vi "Time lapse wait for next frame.vi"(6 "error in (no error)":errorcluster, 8 "Frame Interval (s)":dbl=1.0, 9 "Time of last frame in":u32) -> (0 "error out":errorcluster, 1 "Stopped?":bool, 2 "Sec. till next frame":ext(slide), 3 "Time of this frame out (ms)":u32)   [LabVIEW 2016]
doc: "Waits for the specified time. Used in time-lapse data acquisition."
uses:
  Autofocus Globals.vi
panel:
  in  "Go now":bool
  in  "Pause":bool
  in  "Stop":bool
  # "Parameters not for interactive use"
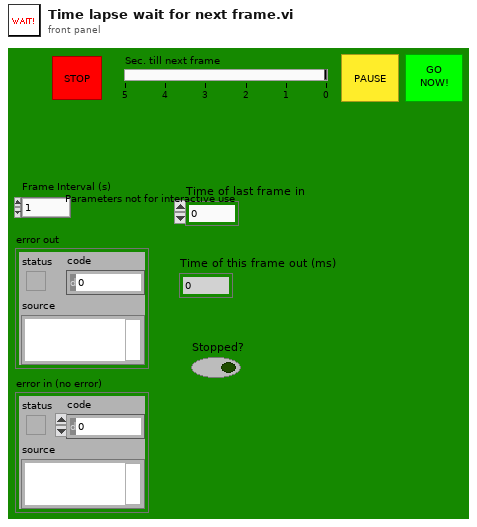
[diagram p1: front panel]
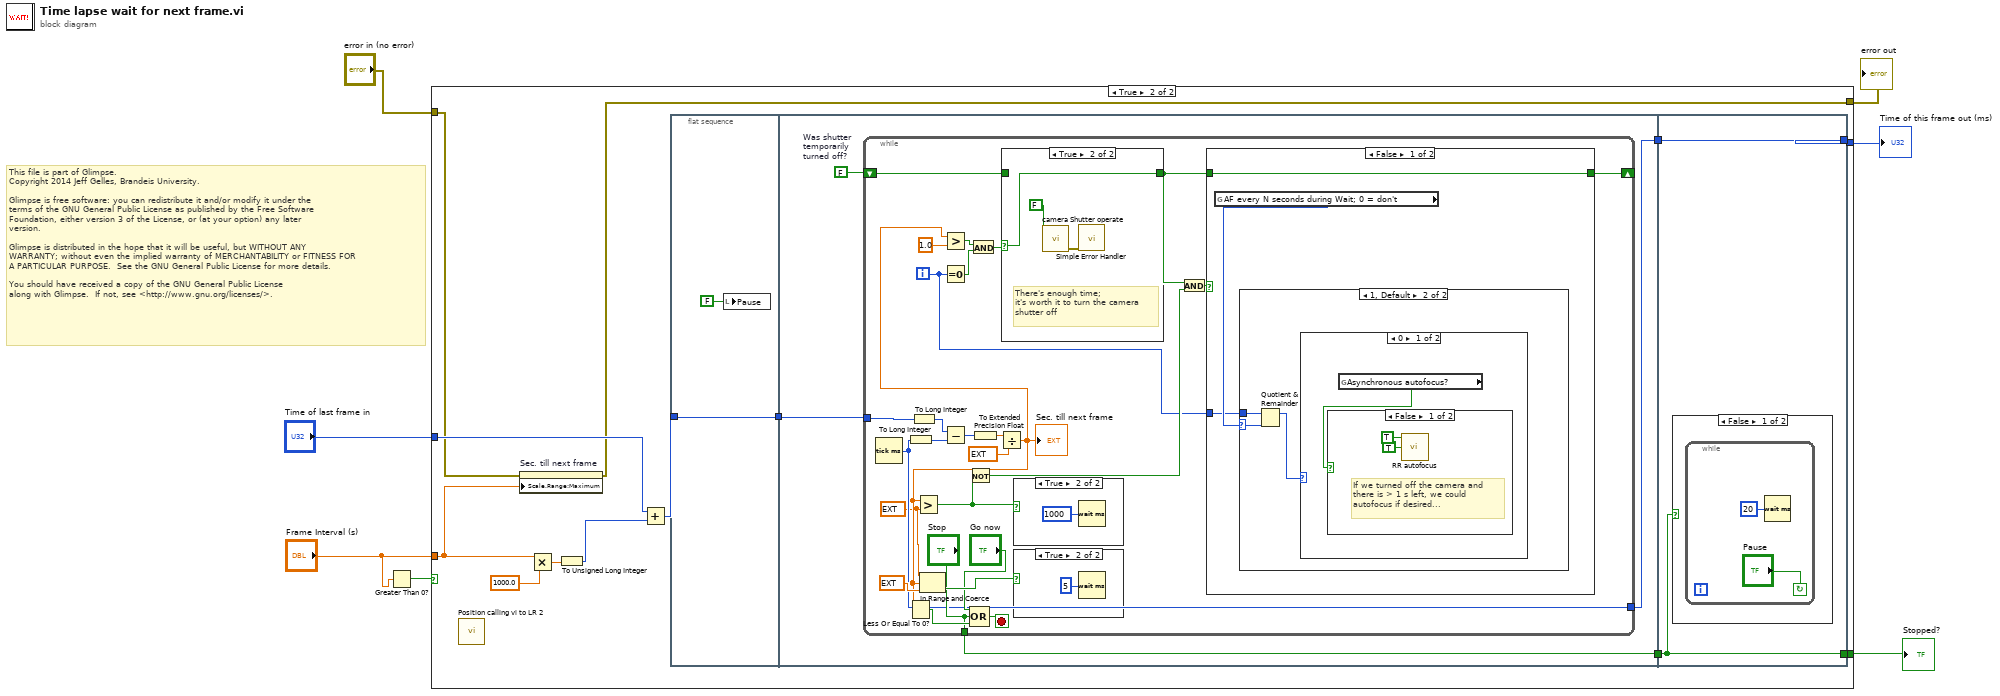
[diagram p0: block diagram]
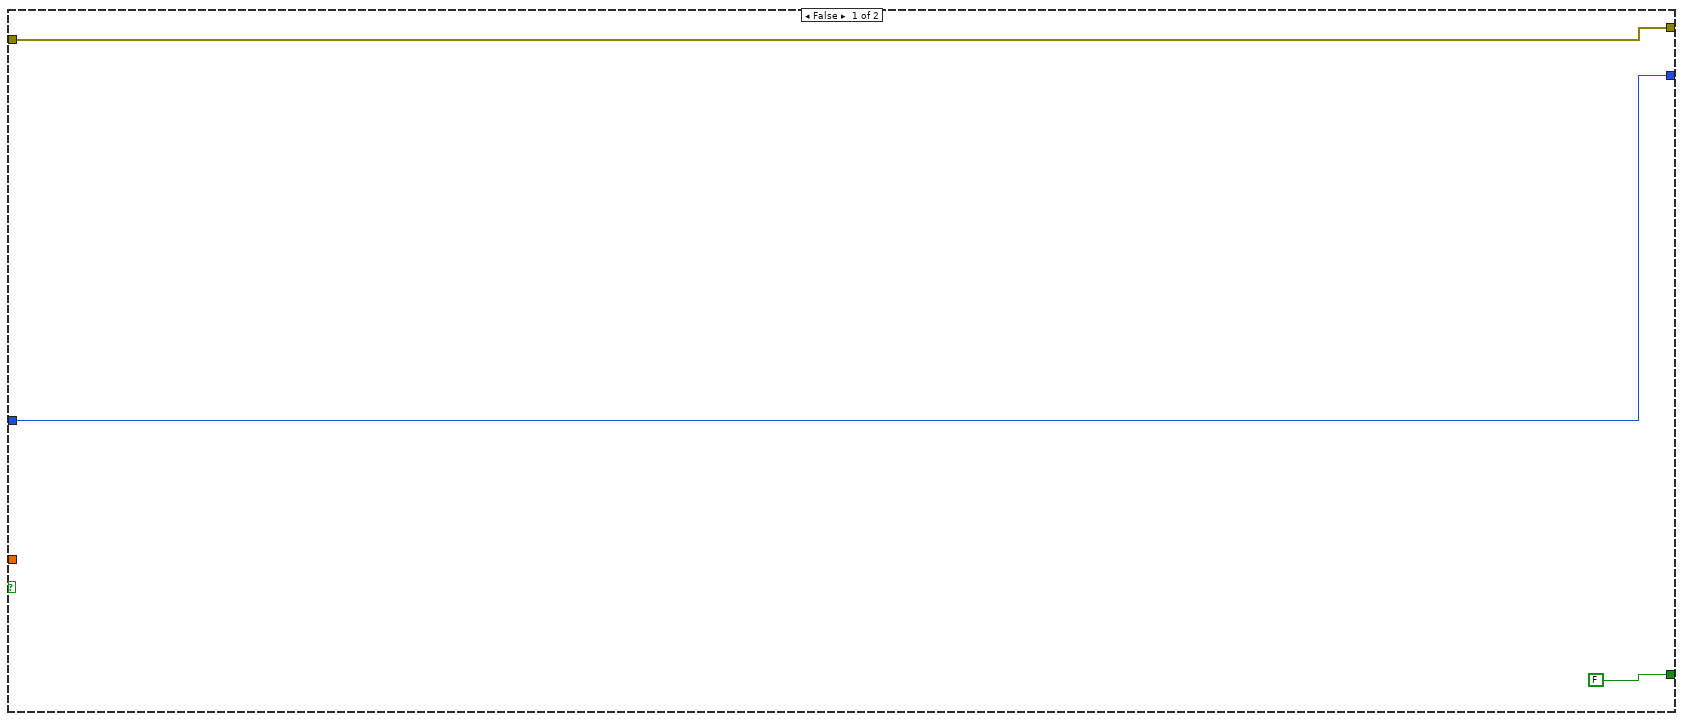
[diagram p2: hidden frame]
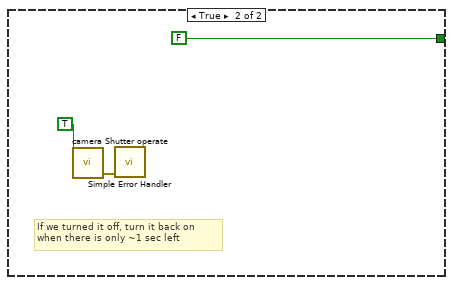
[diagram p6: hidden frame]
diagram:
  # "This file is part of Glimpse. \nCopyright 2014 Jeff Gelles, Brandeis University.    \n\nGlimpse is free software: you can redistribute it and/or modify it under the \nterms of the GNU General Public License as published by the Free Software \nFoundation, either version 3 of the License, or (at your option) any later \nversion.\n\nGlimpse is distributed in the hope that it will be useful, but WITHOUT ANY \nWARRANTY; without even the implied warranty of MERCHANTABILITY or FITNESS FOR \nA PARTICULAR PURPOSE.  See the GNU General Public License for more details.\n\nYou should have received a copy of the GNU General Public License\nalong with Glimpse.  If not, see <http://www.gnu.org/licenses/>."
  n1 = Greater Than 0?(x="Frame Interval (s)") -> (x > 0?=w3:bool)
  n2 = case shown="True" w3 {
    tunnel: [FALSE w23] -> w7
    tunnel: [w9 w22] -> w6
    tunnel: "Time of last frame in" -> [w9 w19]
    tunnel: "Frame Interval (s)" -> [_ w16]
    tunnel: [w8 w15] -> w2
    tunnel: "error in (no error)" -> [w8 w14]
    frame False {
    }
    frame True {
      n3 = call "Position calling vi to LR 2.vi"() -> ()  [unwired: 2 in, 4 out]
      n4 = property on="Sec. till next frame" class="Slide (strict)"(error in=w14, "Scale.Range:Maximum"=w16) -> (error out=w15:errorcluster)  [unwired: 1 in, 1 out]
      n5 = Multiply(x=w16, y=1000.0) -> (x*y=w20:dbl)
      n6 = To Unsigned Long Integer(number=w20) -> (unsigned 32bit integer=w17:u32)
      n7 = Add(x=w19, y=w17) -> (x+y=w18:u32)
      n8 = flat-sequence {
        tunnel: w18 -> [w25]
        tunnel: [w25] -> w11
        tunnel: [w29] -> w13
        tunnel: [w28] -> w12
        tunnel: w11 -> [w27]
        tunnel: [w75] -> w22
        tunnel: [w74] -> w23
        tunnel: w13 -> [w74]
        tunnel: w12 -> [w75]
        frame #0 {
          n9 = local write "Pause"(FALSE ("Pause")) -> ()
        }
        frame #1 {
          w26 = FALSE  # Was shutter temporarily turned off?
          n10 = while {
            tunnel: w27 -> [w55]
            tunnel: [w45] -> w28
            tunnel: ["Stop"] -> w29
            shift-right: [w36] -> _
            shift-left: w26 -> [w40]
            i -> [w30]
            stop <- w49 stop-if-true
            w33 = ext 1.04999999999999999996 ("y")
            n11 = Tick Count (ms)() -> (millisecond timer value=w45:u32)
            n12 = To Long Integer(number=w45) -> (32bit integer=w32:i32)
            n13 = To Long Integer(number=w55) -> (32bit integer=w31:i32)
            n14 = Equal To 0?(x=w30) -> (x = 0?=w42:bool)
            n15 = Subtract(x=w31, y=w32) -> (x-y=w54:i32)
            n16 = To Extended Precision Float(1:w54) -> (0:w53:ext)
            n17 = Divide(x=w53, y=ext 1000.0) -> (x/y=w34:ext)
            "Sec. till next frame" <- w34
            n18 = Less Or Equal To 0?(x=w34) -> (x <= 0?=w48:bool)
            n19 = Greater?(x=w34, y=w33) -> (0:w38:bool)
            n20 = In Range and Coerce(upper limit=w33, x=w34, lower limit=ext 0.01 ("y")) -> (In Range?=w50:bool)  [unwired: 1 out]
            n21 = Greater?(x=w34, y=1.0) -> (0:w43:bool)
            n22 = Not(x=w38) -> (.not. x?=w37:bool)
            n23 = Compound Arithmetic op=OR("Go now", "Stop", w48) -> (w49:bool)
            n24 = And(x=w43, y=w42) -> (x .and. y?=w41:bool)
            n25 = case shown="True" w41 {
              selector: w41 -> [_ w71]
              tunnel: [w68 w71] -> w35
              tunnel: w40 -> [w68 _]
              frame False {
              }
              frame True {
                # "There's enough time;\nit's worth it to turn the camera\nshutter off"
                n26 = call "camera Shutter operate.vi"("Open?"=FALSE) -> ("error out"=w69:errorcluster)  [unwired: 1 in, 6 out]
                n27 = call <vilib>:"Simple Error Handler.vi"("error in (no error)"=w69) -> ()  [unwired: 1 in, 8 out]
              }
            }
            n28 = case shown="True" w38 {
              frame False {
              }
              frame True {
                n29 = Wait (ms)(milliseconds to wait=u32 1000) -> ()  [unwired: 1 out]
              }
            }
            n30 = case shown="True" w50 {
              frame False {
              }
              frame True {
                n31 = Wait (ms)(milliseconds to wait=u32 5) -> ()  [unwired: 1 out]
              }
            }
            n32 = And(x=w35, y=w37) -> (x .and. y?=w39:bool)
            n33 = case shown="False" w39 {
              tunnel: w35 -> [w58 _]
              tunnel: [w58 FALSE ("Shutter turned off?")] -> w36
              tunnel: w30 -> [w56 _]
              frame False {
                n34 = global read "Autofocus Globals.vi" "AF every N seconds during Wait; 0 = don't"() -> (w57:u16)
                n35 = case shown="1, Default" w57 {
                  selector: w57 -> [_ w61]
                  tunnel: w56 -> [_ w60]
                  frame 0 {
                  }
                  frame 1, Default {
                    n36 = Quotient & Remainder(x=w60, y=w61) -> (x-y*floor(x/y)=w59:i32)  [unwired: 1 out]
                    n37 = case shown="0" w59 {
                      frame 0 {
                        n38 = global read "Autofocus Globals.vi" "Asynchronous autofocus?"() -> (w62:bool)
                        n39 = case shown="False" w62 {
                          frame False {
                            # "If we turned off the camera and\nthere is > 1 s left, we could \nautofocus if desired..."
                            n40 = call "RR autofocus.vi"("Close camera shutter during autofocus?"=TRUE, "Close laser shutter when autofocus is done?"=TRUE) -> ()  [unwired: 5 in, 1 out]
                          }
                          frame True {
                          }
                        }
                      }
                      frame 1, Default {
                      }
                    }
                  }
                }
              }
              frame True {
                # "If we turned it off, turn it back on \nwhen there is only ~1 sec left"
                n41 = call "camera Shutter operate.vi"("Open?"=TRUE) -> ("error out"=w66:errorcluster)  [unwired: 1 in, 6 out]
                n42 = call <vilib>:"Simple Error Handler.vi"("error in (no error)"=w66) -> ()  [unwired: 1 in, 8 out]
              }
            }
          }
        }
        frame #2 {
          n43 = case shown="False" w74 {
            frame False {
              n44 = while {
                stop <- "Pause" continue-if-true
                n45 = Wait (ms)(milliseconds to wait=u32 20) -> ()  [unwired: 1 out]
              }
            }
            frame True {
            }
          }
        }
      }
    }
  }
  "Stopped?" <- w7
  "Time of this frame out (ms)" <- w6
  "error out" <- w2
